vi "Configure Current Limit.vi"(7 "Behavior (0: Regulate)":u16(ring) items=["Regulate", "Trip"], 8 "error in (no error)":errorcluster, 9 "Current Limit (5.0 A)":dbl=5.0 caption="Current Limit (5 A)" format="%.2f", 10 "Channel (0: 30V Channel)":T1 caption="Channel (0: +6V)" items=["30V/3A Channel", "30V/3A Channel", "5V/3A Channel"], 11 "VISA resource name":refnum<visa-resource-name>) -> (0 "error out":errorcluster, 3 "VISA resource name out":refnum<visa-resource-name>)   [LabVIEW 2015, in "RIGOL DP800 Series.lvlib"]
doc: "Configures over current protection (OCP). Specify the output current limit value and the behavior of the power supply when the output current is greater than or equal to that value."
uses:
  <instrlib>/RIGOL DP800 Series/RIGOL DP800 Series.lvlib
  <instrlib>/RIGOL DP800 Series/Public/Channels.ctl
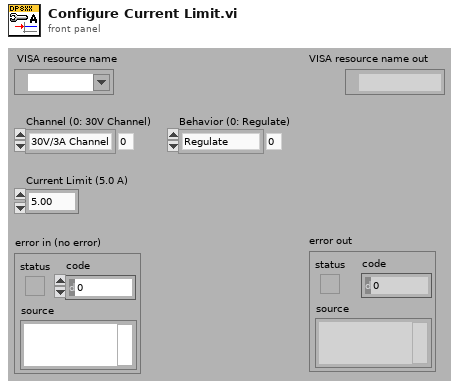
[diagram p1: front panel]
types:
  T1 = typedef "RIGOL DP800 Series.lvlib/Channels.ctl" = i32
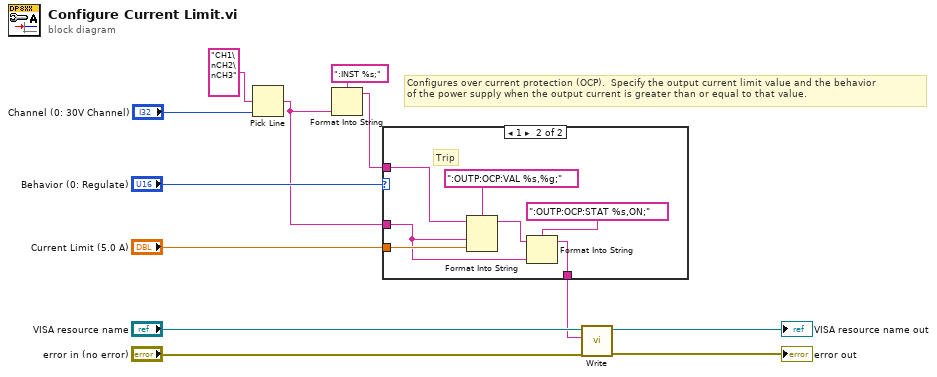
[diagram p0: block diagram]
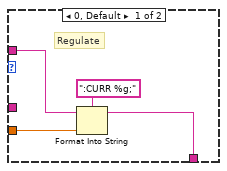
[diagram p2: hidden frame]
diagram:
  # "Configures over current protection (OCP).  Specify the output current limit value and the behavior \nof the power supply when the output current is greater than or equal to that value."
  n1 = Pick Line(multi-line string="CH1\nCH2\nCH3", line index="Channel (0: 30V Channel)") -> (output string=w7:string)  [unwired: 1 in]
  n2 = Format Into String(format string=":INST %s;", w7) -> (resulting string=w8:string)  [unwired: 2 in, 1 out]
  n3 = case shown="1" "Behavior (0: Regulate)" {
    tunnel: "Current Limit (5.0 A)" -> [w15 w22]
    tunnel: w8 -> [w14 w21]
    tunnel: [w13 w19] -> w2
    tunnel: w7 -> [_ w18]
    frame 0, Default {
      # "Regulate"
      n4 = Format Into String(format string=":CURR %g;", initial string=w14, w15) -> (resulting string=w13:string)  [unwired: 1 in, 1 out]
    }
    frame 1 {
      # "Trip"
      n5 = Format Into String(format string=":OUTP:OCP:VAL %s,%g;", initial string=w21, w18, w22) -> (resulting string=w20:string)  [unwired: 1 in, 1 out]
      n6 = Format Into String(format string=":OUTP:OCP:STAT %s,ON;", initial string=w20, w18) -> (resulting string=w19:string)  [unwired: 1 in, 1 out]
    }
  }
  n7 = call <instrlib>:"Write.vi"("error in (no error)"="error in (no error)", "Write Buffer (\"\")"=w2, "VISA resource name"="VISA resource name") -> ("error out"=→"error out":errorcluster, "VISA resource name out"=→"VISA resource name out":refnum<visa-resource-name>)  [unwired: 7 in]
